vi "File Size Rollover_Log Record Exceeds Threshold.vi"() -> ()   [LabVIEW 2018]
uses:
  src/api/logger_class/Log Levels.ctl
  src/api/configuration/formatters/format_string_formatter/Format String.lvclass
  C:/Users/Colin/Documents/software_projects/labview/glog/src/api/extension/formatter_interface/Formatter.lvclass
  src/api/configuration/handlers/file_handler/File Handler.lvclass
  C:/Users/Colin/Documents/software_projects/labview/glog/src/api/extension/formatting_handler_interface/Formatting Handler.lvclass
  src/api/logger_class/Log (Parts).vi
  src/api/logger_class/Logger.lvclass
panel:
  out "3 files?":bool caption="1 file? (1st)"
  out "2 files?":bool caption="1 file? (1st)"
  in  "delete when done?":bool=TRUE
  out "error out":errorcluster
  out "1 file?":bool caption="1 file? (1st)"
  # "Locals"
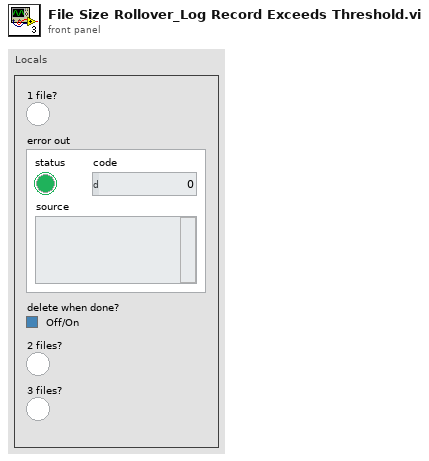
[diagram p1: front panel]
types:
  T1 = typedef "GLog.lvlib/Logger.lvclass/Log Levels.ctl" = enum16{"Trace", "Debug", "Info", "Warning", "Error", "Critical"}
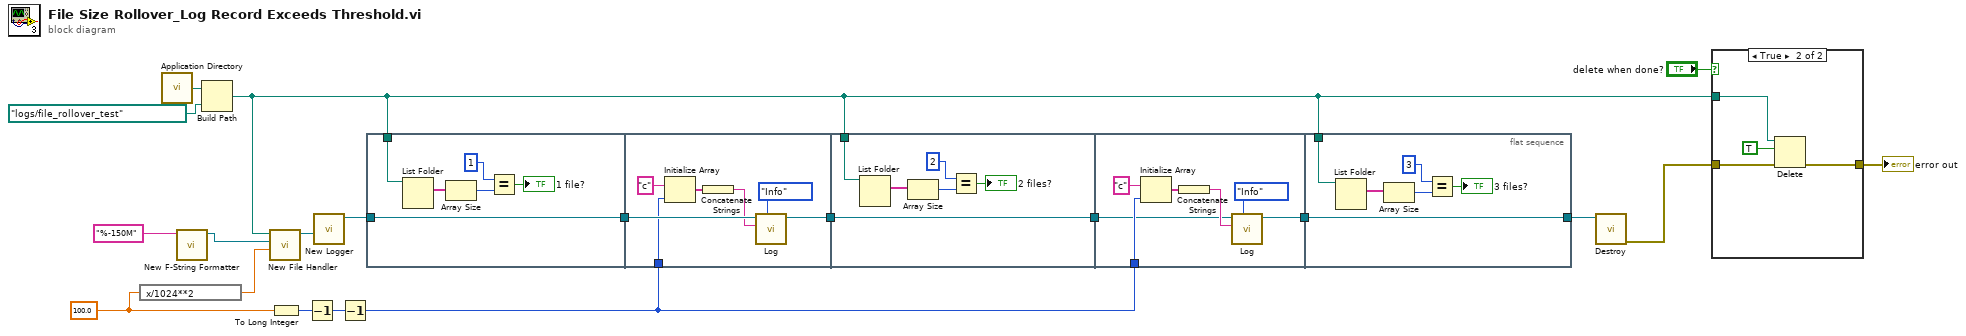
[diagram p0: block diagram]
diagram:
  w11 = 100.0
  n1 = expression code="x/1024**2"(w11) -> (w12:dbl)
  n2 = call <vilib>:"Application Directory.vi"() -> ("Application Directory"=w19:path)
  n3 = call "New F-String Formatter.vi"("format string (\"%T | %L | %M\")"="%-150M" ("format string (\"%T | %L | %M\")")) -> ("new f-string formatter"=w10:refnum<class "Format String.lvclass">)  [unwired: 10 in]
  n4 = Build Path(base path=w19, name or relative path=path "logs/file_rollover_test") -> (appended path=w5:path)
  n5 = call "New File Handler.vi"("max file size [MB](50)"=w12, "formatter (JSON)"=w10, "log directory (<app dir>/logs)"=w5) -> ("file handler"=w20:refnum<class "File Handler.lvclass">)  [unwired: 8 in]
  n6 = To Long Integer(number=w11) -> (32bit integer=w7:i32)
  n7 = Decrement(x=w7) -> (x-1=w3:i32)
  n8 = call "New Logger.vi"("log handler (file handler)"=w20) -> ("logger"=w15:refnum<class "Logger.lvclass">)  [unwired: 9 in, 1 out]
  n9 = Decrement(x=w3) -> (x-1=w2:i32)
  n10 = flat-sequence {
    tunnel: w15 -> [w26]
    tunnel: [w26] -> w14
    tunnel: w5 -> [w22]
    tunnel: [w31] -> w16
    tunnel: w14 -> [w32]
    tunnel: w2 -> [w27]
    tunnel: w5 -> [w39]
    tunnel: w16 -> [w38]
    tunnel: [w38] -> w8
    tunnel: w8 -> [w40]
    tunnel: w2 -> [w41]
    tunnel: [w42] -> w6
    tunnel: [w52] -> w4
    tunnel: w6 -> [w52]
    tunnel: w5 -> [w47]
    frame #0 {
      n11 = List Folder(path=w22) -> (filenames=w23:string[])  [unwired: 3 in, 3 out]
      n12 = Array Size(array=w23) -> (size(s)=w24:i32)
      n13 = Equal?(x=1, y=w24) -> (x = y?=→"1 file?":bool)
    }
    frame #1 {
      n14 = Initialize Array("c" ("message"), w27) -> (w29:string[])
      n15 = Concatenate Strings(w29) -> (w28:string)
      n16 = call-poly "Log.vi"("log level"=Log_Levels."Info" ("level"), "message"=w28, "logger in"=w32) -> ("logger out"=w31:refnum<class "Logger.lvclass">)  [unwired: 8 in]
    }
    frame #2 {
      n17 = List Folder(path=w39) -> (filenames=w34:string[])  [unwired: 3 in, 3 out]
      n18 = Array Size(array=w34) -> (size(s)=w36:i32)
      n19 = Equal?(x=2, y=w36) -> (x = y?=→"2 files?":bool)
    }
    frame #3 {
      n20 = Initialize Array("c" ("message"), w41) -> (w44:string[])
      n21 = Concatenate Strings(w44) -> (w43:string)
      n22 = call-poly "Log.vi"("log level"=Log_Levels."Info" ("level"), "message"=w43, "logger in"=w40) -> ("logger out"=w42:refnum<class "Logger.lvclass">)  [unwired: 8 in]
    }
    frame #4 {
      n23 = List Folder(path=w47) -> (filenames=w48:string[])  [unwired: 3 in, 3 out]
      n24 = Array Size(array=w48) -> (size(s)=w50:i32)
      n25 = Equal?(x=3, y=w50) -> (x = y?=→"3 files?":bool)
    }
  }
  n26 = call "Destroy.vi"("logger in"=w4) -> ("error out"=w1:errorcluster)  [unwired: 9 in, 1 out]
  n27 = case shown="True" "delete when done?" {
    tunnel: w5 -> [_ w55]
    tunnel: [_ w54] -> w18
    tunnel: w1 -> [_ w53]
    frame False {
    }
    frame True {
      n28 = Delete(path (use dialog)=w55, entire hierarchy (F)=TRUE, error in=w53) -> (error out=w54:errorcluster)  [unwired: 2 in, 2 out]
    }
  }
  "error out" <- w18
